vi "3KantVip_SubVI.vi"() -> ()   [LabVIEW 2018]
panel:
  in  "Antal iterationer pr. stepper":i32=10
  out "Direction":bool
  out "Enable 3":bool
  out "Enable 2":bool
  out "Enable 1":bool
  in  "stop":bool
  in  "BUND!":bool
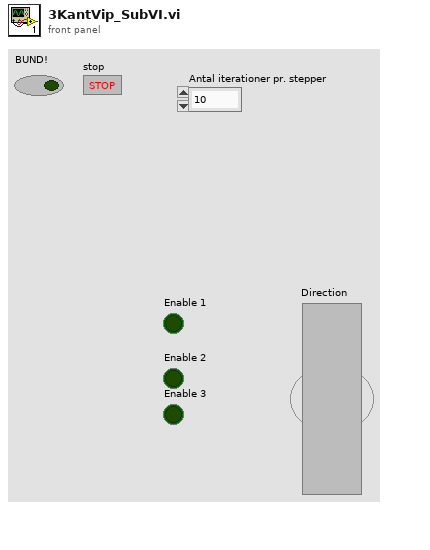
[diagram p1: front panel]
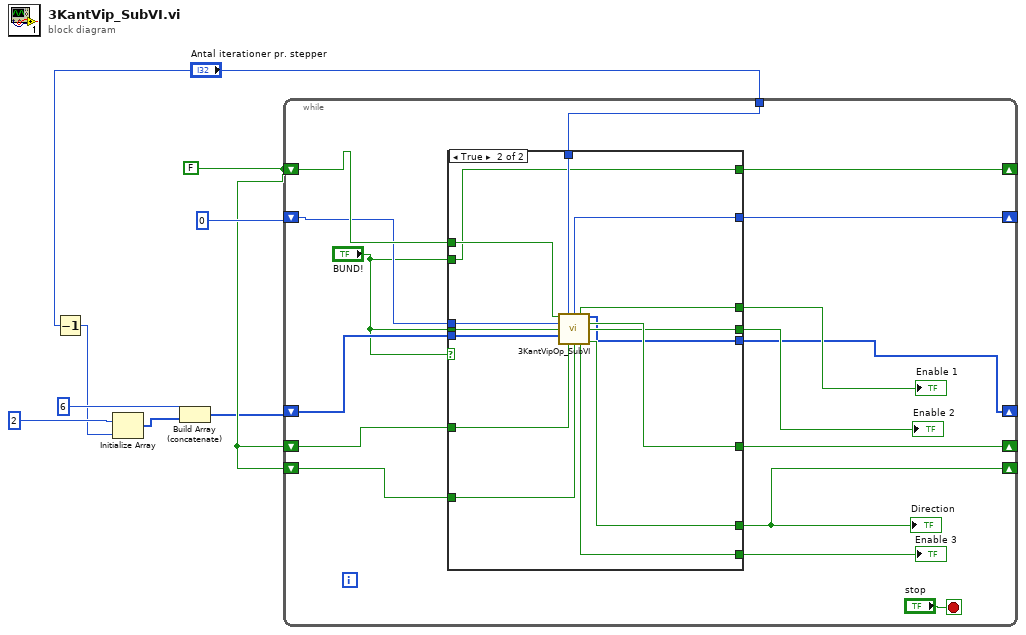
[diagram p0: block diagram]
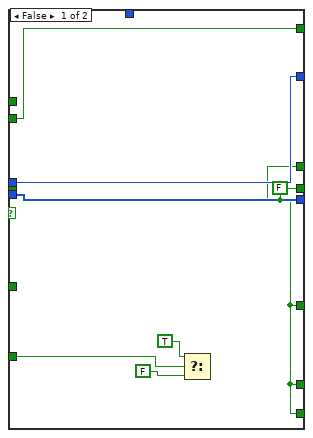
[diagram p2: hidden frame]
diagram:
  w7 = FALSE ("BUND!")
  n1 = Decrement(x="Antal iterationer pr. stepper") -> (x-1=w2:i32)
  n2 = Initialize Array(2, w2) -> (w4:i32[])
  n3 = Build Array (concatenate)(6, w4) -> (w5:i32[])
  n4 = while {
    shift-right: [w10] -> _
    shift-left: w7 -> [w16]
    shift-right: [w23] -> _
    shift-left: w7 -> [w13]
    shift-right: [w22] -> _
    shift-left: 0 -> [w15]
    shift-right: [w9] -> _
    shift-left: w7 -> [w12]
    shift-right: [w18] -> _
    shift-left: w5 -> [w14]
    tunnel: "Antal iterationer pr. stepper" -> [w17]
    stop <- "stop" stop-if-true
    n5 = case shown="True" "BUND!" {
      tunnel: [w25 w46] -> w23
      tunnel: [w30 w45] -> w22
      tunnel: [w25 w44] -> w9
      tunnel: [w25 w43] -> w21
      tunnel: [w25 w42] -> w20
      tunnel: [w25 w41] -> w19
      tunnel: [w29 w40] -> w18
      tunnel: w17 -> [_ w39]
      tunnel: "BUND!" -> [_ w38]
      tunnel: w16 -> [_ w37]
      tunnel: w15 -> [w30 w36]
      tunnel: w14 -> [w29 w35]
      tunnel: w13 -> [_ w34]
      tunnel: w12 -> [w26 w33]
      tunnel: "BUND!" -> [w31 w32]
      tunnel: [w31 w32] -> w10
      frame False {
        w25 = FALSE ("Enable 2")
        n6 = Select(t=TRUE, s=w26, f=FALSE) -> ()  [unwired: 1 out]
      }
      frame True {
        n7 = call "3KantVipOp_SubVI.vi"("Shift 1 in"=w37, "Antal iterationer pr. stepper"=w39, "Loops shift in"=w36, "BUND!"=w38, "Index step array shift in"=w35, "Shift 2 in"=w34, "Direction shift in"=w33) -> ("Loops shift out"=w45:i32, "Enable 1"=w43:bool, "Index step array shift ud"=w40:i32[], "Shift 2 ud"=w46:bool, "Enable 2"=w41:bool, "Enable 3"=w42:bool, "Direction shift ud"=w44:bool)  [unwired: 1 in, 1 out]
      }
    }
    "Enable 1" <- w21
    "Enable 2" <- w19
    "Enable 3" <- w20
    "Direction" <- w9
  }
